vi "HTML_ArrayToPropertyAndValueString.vi"(7 "use a space inbetween prop and value? (T)":bool=TRUE, 10 "Table css-Attributes[]":string[][](array[string])=[["width", "100%"]]) -> (2 "spreadsheet string":string)   [LabVIEW 2014]
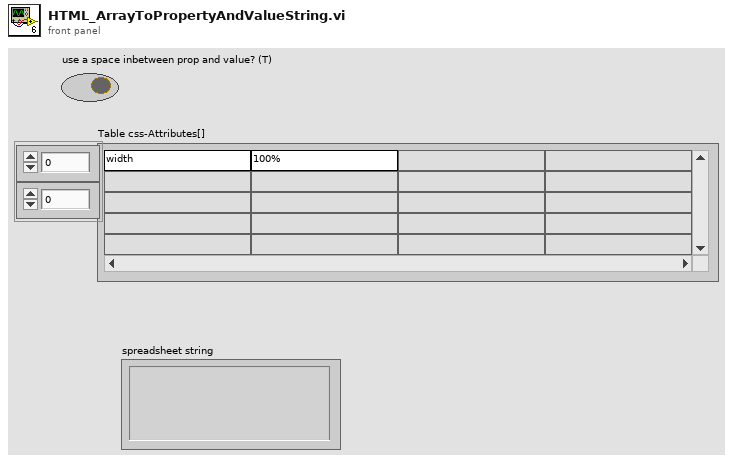
[diagram p1: front panel]
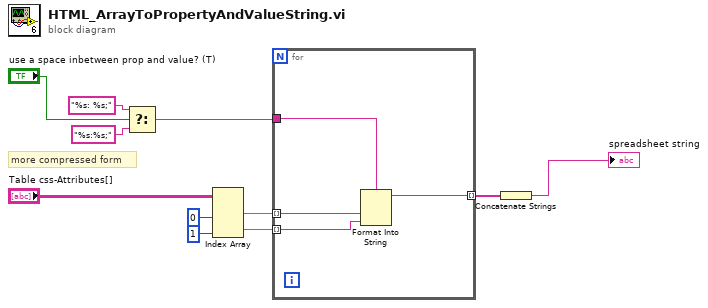
[diagram p0: block diagram]
diagram:
  # "more compressed form"
  n1 = Select(t="%s: %s;" ("format string"), s="use a space inbetween prop and value? (T)", f="%s:%s;" ("format string")) -> (s? t:f=w1:string)
  n2 = Index Array(array="Table css-Attributes[]", index (col) #1=0 ("disabled index (col)"), index (col) #2=1 ("index (col)")) -> (element #1=w10:string[], element #2=w9:string[])  [unwired: 2 in]
  n3 = for {
    tunnel: w10 -> [w15] mode=indexing
    tunnel: w9 -> [w14] mode=indexing
    tunnel: [w13] -> w6 mode=indexing
    tunnel: w1 -> [w12]
    n4 = Format Into String(format string=w12, w15, w14) -> (resulting string=w13:string)  [unwired: 2 in, 1 out]
  }
  n5 = Concatenate Strings(w6) -> (→"spreadsheet string":string)
